vi "NI VeriStand - Search for Item by Name.vi"(8 "error in":errorcluster, 10 "Item Name":string, 11 "Section Ref in":T1 format="%.0x") -> (0 "error out":errorcluster, 2 "Item Ref":T1 format="%.0x", 3 "Section Ref out":T1 format="%.0x", 4 "Found":bool)   [LabVIEW 2020, in "Custom Device Utility Library.lvlib"]
doc: "Searches a custom device section for the item(s) you specify. You can search for one or multiple items by name, GUID, or property name and value. You must manually select the polymorphic instance to use."
uses:
  <vilib>/NI VeriStand/Custom Device Tools/Custom Device Utility Library/Custom Device Utility Library.lvlib
  <vilib>/NI VeriStand/Custom Device API/Custom Device Item Ref.ctl
  <vilib>/NI VeriStand/Custom Device Tools/Custom Device Utility Library/NI VeriStand - Ref Constants.vi
  <vilib>/NI VeriStand/Custom Device API/Custom Device API.lvlib
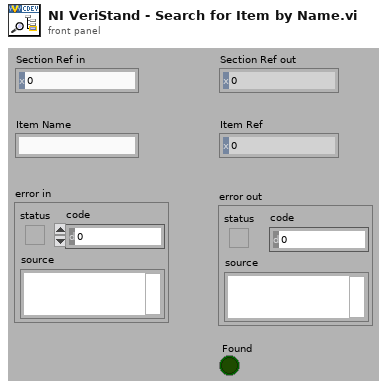
[diagram p1: front panel]
types:
  T1 = typedef "Custom Device API.lvlib/Custom Device Item Ref.ctl" = u64
  T2 = typedef "Custom Device API.lvlib/Custom Device Item Info.ctl" = cluster{"Name":string, "Is Channel":bool, "GUID":string, "Is Waveform":bool}
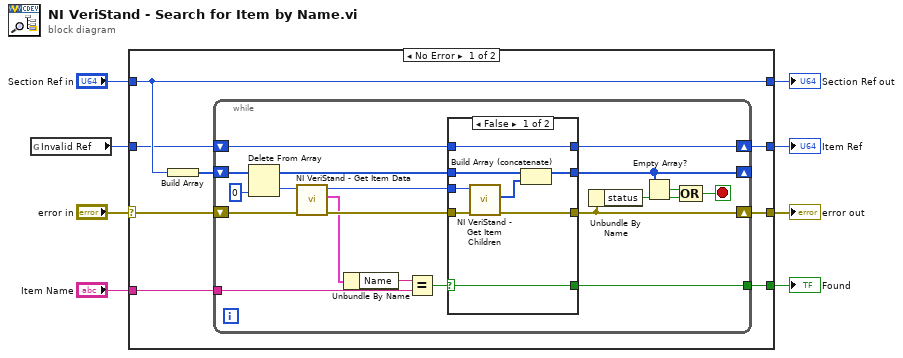
[diagram p0: block diagram]
diagram:
  n1 = global read "NI VeriStand - Ref Constants.vi" "Invalid Ref"() -> (w1:T1)
  n2 = case shown="No Error" "error in" {
    selector: "error in" -> [w11 w48]
    tunnel: "Section Ref in" -> [w12 w49]
    tunnel: "Item Name" -> [w15 _]
    tunnel: [w14 w48] -> w6
    tunnel: [w13 _] -> w5
    tunnel: [w10 w47] -> w4
    tunnel: [w12 w49] -> w3
    tunnel: w1 -> [w9 w47]
    frame No Error {
      n3 = Build Array(w12) -> (w16:T1[])
      n4 = while {
        shift-right: [w19] -> w14
        shift-left: w11 -> [w34]
        shift-right: [w18] -> _
        shift-left: w16 -> [w33]
        tunnel: w15 -> [w29]
        tunnel: [w24] -> w13
        shift-right: [w26] -> w10
        shift-left: w9 -> [w23]
        stop <- w20 stop-if-true
        n5 = Delete From Array(array=w33, index=0) -> (deleted portion=w31:T1, array with subset deleted=w27:T1[])  [unwired: 1 in]
        n6 = call <vilib>:"NI VeriStand - Get Item Data.vi"("error in (no error)"=w34, "Item Ref in"=w31) -> ("error out"=w35:errorcluster, "Item Info"=w30:T2, "Item Ref out"=w28:T1)  [unwired: 7 out]
        n7 = Unbundle By Name(w30) -> ("Name"=w17:string)
        n8 = Equal?(x=w17, y=w29) -> (x = y?=w25:bool)
        n9 = case shown="False" w25 {
          selector: w25 -> [w37 w45]
          tunnel: [w43 w46] -> w19
          tunnel: w35 -> [w42 w46]
          tunnel: w28 -> [w41 w44]
          tunnel: w27 -> [w40 _]
          tunnel: [w38 _] -> w18
          tunnel: [w36 w44] -> w26
          tunnel: [w37 w45] -> w24
          tunnel: w23 -> [w36 _]
          frame False {
            n10 = call <vilib>:"NI VeriStand - Get Item Children.vi"("error in (no error)"=w42, "Item Ref in"=w41) -> ("error out"=w43:errorcluster, "Child Refs"=w39:T1[])  [unwired: 8 out]
            n11 = Build Array (concatenate)(w40, w39) -> (w38:T1[])
          }
          frame True {
          }
        }
        n12 = Unbundle By Name(w19) -> ("status"=w21:bool)
        n13 = Empty Array?(array=w18) -> (empty?=w22:bool)
        n14 = Compound Arithmetic op=OR(w22, w21) -> (w20:bool)
      }
    }
    frame Error {
    }
  }
  "Found" <- w5
  "error out" <- w6
  "Section Ref out" <- w3
  "Item Ref" <- w4
